vi "8164B Set Attenuation (1).vi"(8 "error in":errorcluster, 10 "Att 1, dB":dbl=40.0 format="%#_13g", 11 "KeySight 8164B control in":T1) -> (0 "error out":errorcluster, 3 "KeySight 8164B control out":T1)   [LabVIEW 2018, in "KeySight 8164B LAN InstrLib.lvlib"]
uses:
  KeySight 8164B LAN InstrLib.lvlib
  typedefs/KeySight 8164B control.ctl
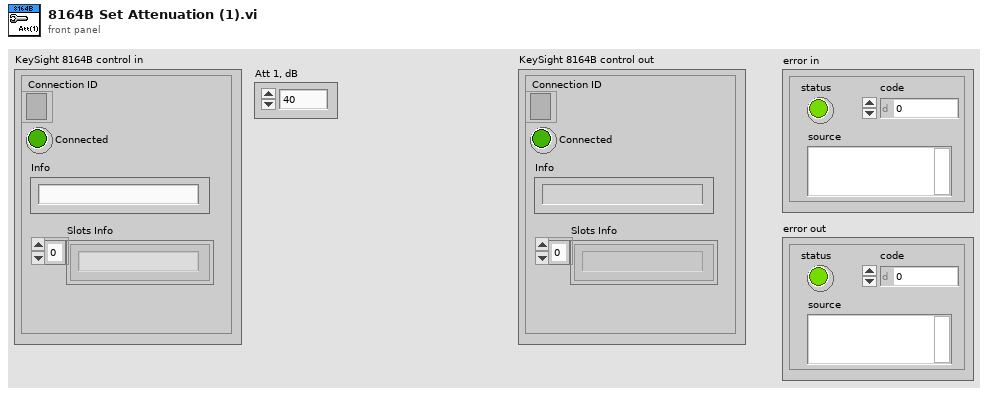
[diagram p1: front panel]
types:
  T1 = typedef "KeySight 8164B LAN InstrLib.lvlib/KeySight 8164B control.ctl" = cluster{"Connection ID":refnum<k5>, "Connected":bool, "Info":string, "Slots Info":string[]}
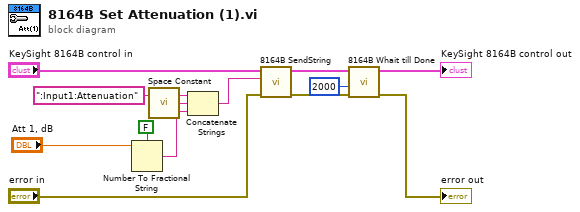
[diagram p0: block diagram]
diagram:
  n1 = Number To Fractional String(use system decimal point (T)=FALSE, number="Att 1, dB") -> (F-format string=w1:string)  [unwired: 2 in]
  n2 = call <vilib>:"Space Constant.vi"() -> ("String"=w4:string)
  n3 = Concatenate Strings(":Input1:Attenuation", w4, w1) -> (w3:string)
  n4 = call "8164B SendString.vi"("error in"="error in", "CMD"=w3, "KeySight 8164B control in"="KeySight 8164B control in") -> ("error out"=w7:errorcluster, "KeySight 8164B control out"=w9:T1)  [unwired: 7 in]
  n5 = call "8164B Whait till Done.vi"("error in"=w7, "timeout ms"=2000, "KeySight 8164B control in"=w9) -> ("error out"=→"error out":errorcluster, "KeySight 8164B control out"=→"KeySight 8164B control out":T1)  [unwired: 7 in]
